vi "Destroy Events.vi"(8 "error in (no error)":errorcluster, 11 "Execution Events":T1) -> ()   [LabVIEW 2022 SP3, in "FlexBlocks Support.lvlib"]
uses:
  FlexBlocks Support.lvlib
  Block State.ctl
  Block Phase.ctl
  Block Status.ctl
  Block Status with Error.ctl
  Block Command.ctl
  Worker Block.ctl
  Worker Registration.ctl
  Execution Events.ctl
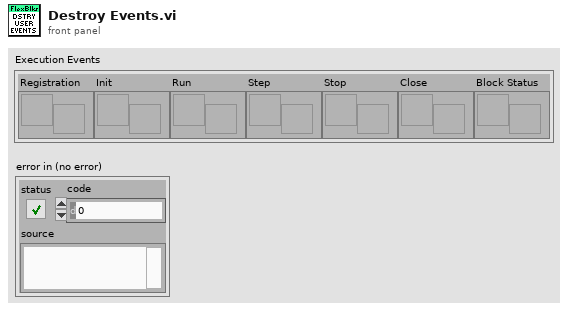
[diagram p1: front panel]
types:
  T1 = typedef "FlexBlocks Support.lvlib/Execution Events.ctl" = cluster{"Registration":refnum<user-event>, "Init":refnum<user-event>, "Run":refnum<user-event>, "Step":refnum<user-event>, "Stop":refnum<user-event>, "Close":refnum<user-event>, "Block Status":refnum<user-event>}
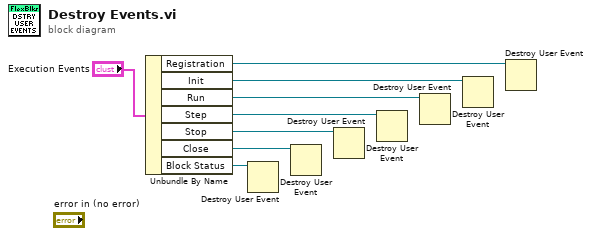
[diagram p0: block diagram]
diagram:
  n1 = Unbundle By Name("Execution Events") -> ("Registration"=w1:refnum<user-event>, "Init"=w2:refnum<user-event>, "Run"=w3:refnum<user-event>, "Step"=w4:refnum<user-event>, "Stop"=w5:refnum<user-event>, "Close"=w6:refnum<user-event>, "Block Status"=w7:refnum<user-event>)
  n2 = Destroy User Event(user event=w7) -> ()  [unwired: 1 in, 1 out]
  n3 = Destroy User Event(user event=w6) -> ()  [unwired: 1 in, 1 out]
  n4 = Destroy User Event(user event=w5) -> ()  [unwired: 1 in, 1 out]
  n5 = Destroy User Event(user event=w4) -> ()  [unwired: 1 in, 1 out]
  n6 = Destroy User Event(user event=w3) -> ()  [unwired: 1 in, 1 out]
  n7 = Destroy User Event(user event=w2) -> ()  [unwired: 1 in, 1 out]
  n8 = Destroy User Event(user event=w1) -> ()  [unwired: 1 in, 1 out]
